vi "Main.vi"() -> ()   [LabVIEW 2017]
doc: "Use this template to build a user interface event handler design pattern. Use this pattern for dialog boxes and other user interfaces. You also can create and execute user-defined events that the VI can handle the same way as user interface events."
panel:
  in  "Exit":bool
  in  "Log In":bool
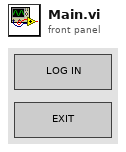
[diagram p1: front panel]
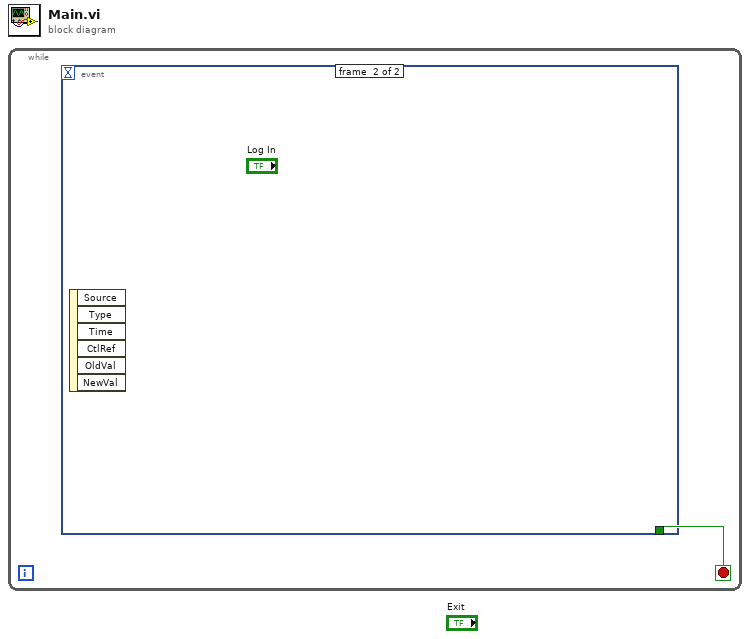
[diagram p0: block diagram]
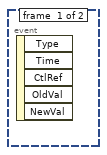
[diagram p2: hidden frame]
diagram:
  n1 = while {
    stop <- w1 stop-if-true
    n2 = event {
      selector: _ -> [_ _]
      dyn-events: _ -> [_ _]
      timeout: _ -> [_ _]
      tunnel: [_ _] -> w1
      event #0 {
        n3 = event-data() -> ()  [unwired: 1 in, 5 out]
      }
      event #1 {
        n4 = event-data() -> ()  [unwired: 1 in, 6 out]
      }
    }
  }
